vi "CreatePrivateEvents.vi"(8 "error in (no error)":errorcluster, 11 "JKI.Robot.SMO":refnum<class "JKI.Robot.SMO.lvclass">) -> (0 "error out":errorcluster, 3 "JKI.Robot.SMO out":refnum<class "JKI.Robot.SMO.lvclass">)   [LabVIEW 2014, in "JKI.Robot.SMO.lvclass"]
doc: "---------------------------------------------------------------\nJKI State Machine Objects™\nhttp://jki.net/state-machine-objects/\nCopyright (C) 2005-2015, JKI <info@jki.net>\nALL RIGHTS RESERVEDJKI State Machine Objects (SMO) 1.0.0.4\nJKI - JKI\nCopyright (c) 2015, JKI"
uses:
  JKI.Robot.SMO.lvclass
  JKI.Robot.SMO.lvclass/JKI.Robot.SMO.ctl
  Typedefs/PrivateEvents--JKI.Robot.SMO.SetGrabberPosition.ctl
  Typedefs/PrivateEvents--JKI.Robot.SMO.SetJointRotation.ctl
  Typedefs/JointType--Enum.ctl
  JKI.Robot.SMO.Base/JKI.Robot.SMO.Base.lvclass
panel:
  # "For instructions on how to use the JKI State Machine Objects, examples and video tutorials, visit:\nhttp://jki.net/state-machine-objects/\n\nJKI State Machine Objects™\nhttp://jki.net/state-machine-objects/\nCopyright (C) 2005-2015, JKI <info@jki.net>\nALL RIGHTS RESERVED"
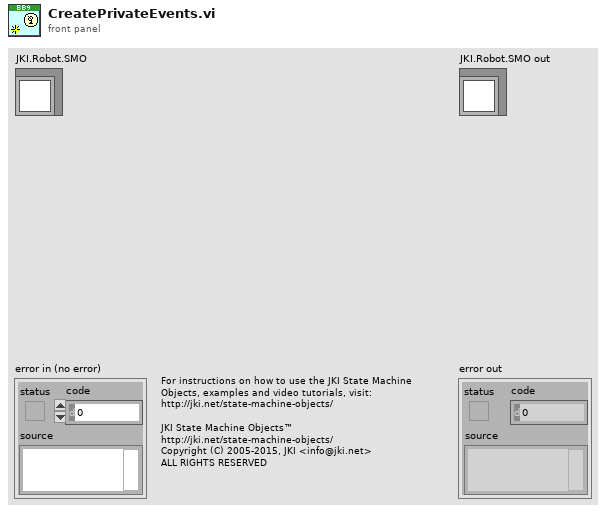
[diagram p1: front panel]
types:
  T1 = typedef "JKI.Robot.SMO.lvclass/PrivateData--Ref.ctl" = refnum<data-value>
  T2 = typedef "JKI.Robot.SMO.lvclass/PrivateEvents--JKI.Robot.SMO.SetJointRotation.ctl" = cluster{"Joint":T3, "Rotation (Deg)":dbl}
  T3 = typedef "JointType--Enum.ctl" = enum16{"A_Shoulder", "B_Elbow", "C_Wrist", "D_Base"}
  T4 = typedef "JKI.Robot.SMO.lvclass/PrivateEvents--JKI.Robot.SMO.SetGrabberPosition.ctl" = dbl
  T5 = typedef "JKI.Robot.SMO.lvclass/PrivateData--Cluster.ctl" = cluster{"Configuration":T6, "Public Events":T7, "Robot Position":T8, "Private Events":T9}
  T6 = typedef "JKI.Robot.SMO.lvclass/Configuration--Cluster.ctl" = cluster{"Suffix":string}
  T7 = typedef "JKI.Robot.SMO.lvclass/PublicEvents--Cluster.ctl" = cluster{"Data Changed":refnum<user-event>}
  T8 = typedef "RobotPosition--Cluster.ctl" = cluster{"Claw%":dbl, "JointA":dbl, "JointB":dbl, "JointC":dbl, "JointD":dbl}
  T9 = typedef "JKI.Robot.SMO.lvclass/PrivateEvents--Cluster.ctl" = cluster{"SetGrabberPosition":refnum<user-event>, "SetJointRotation":refnum<user-event>}
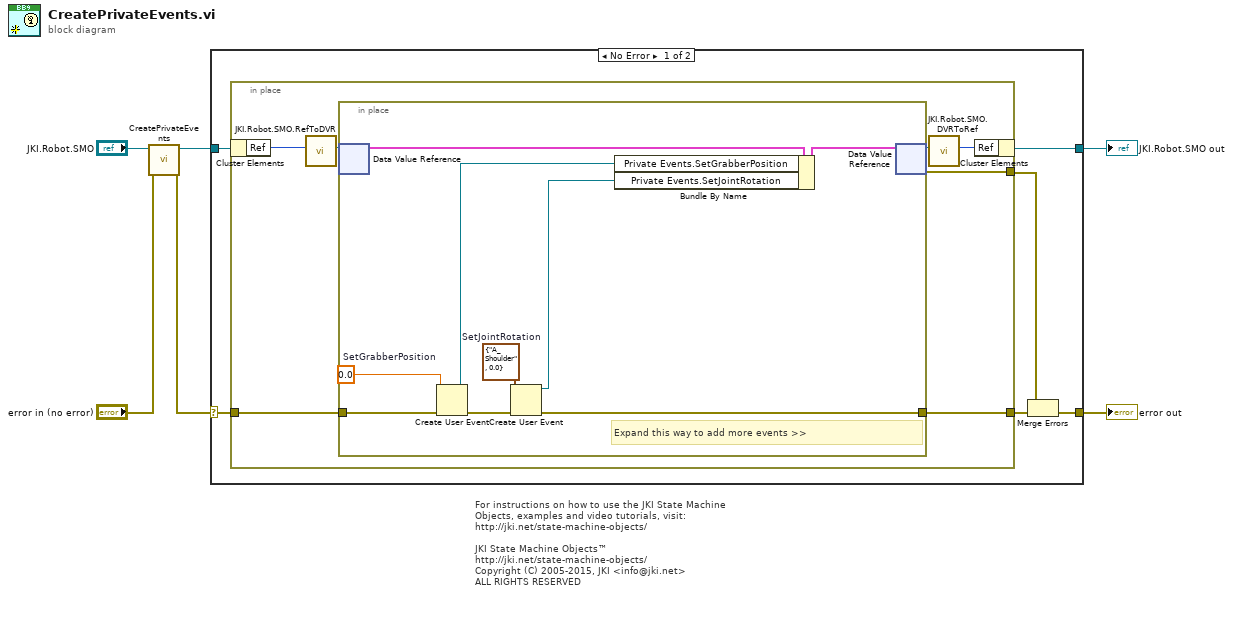
[diagram p0: block diagram]
diagram:
  # "For instructions on how to use the JKI State Machine Objects, examples and video tutorials, visit:\nhttp://jki.net/state-machine-objects/\n\nJKI State Machine Objects™\nhttp://jki.net/state-machine-objects/\nCopyright (C) 2005-2015, JKI <info@jki.net>\nALL RIGHTS RESERVED"
  n1 = call-parent "CreatePrivateEvents.vi"("error in (no error)"="error in (no error)", "SMO"="JKI.Robot.SMO") -> ("error out"=w1:errorcluster, "SMO out"=w3:refnum<class "JKI.Robot.SMO.lvclass">)  [unwired: 8 in]
  n2 = case shown="No Error" w1 {
    selector: w1 -> [w10 w30]
    tunnel: [w8 w30] -> w5
    tunnel: [w11 w29] -> w6
    tunnel: w3 -> [w12 w29]
    frame No Error {
      n3 = in-place {
        in-place-border: w10 -> [w19]
        in-place-border: [w16] -> w7
        in-place-border: [w15] -> w9
        n4 = in-place-cluster #1(w12) -> ("Ref"=w18:u32)
        n5 = call "JKI.Robot.SMO.RefToDVR.vi"("Ref"=w18) -> ("Ref"=w14:T1)  [unwired: 10 in]
        n6 = in-place {
          in-place-border: w19 -> [w28]
          in-place-border: [w22] -> w16
          w21 = T2 {"Joint"=enum."A_Shoulder", "Rotation (Deg)"=0.0}  # SetJointRotation
          w24 = T4 0.0  # SetGrabberPosition
          # "Expand this way to add more events >>"
          n7 = in-place-dvr #2(w14) -> (w27:T5)  [unwired: 1 out]
          n8 = Create User Event(user event datatype=w24, error in=w28) -> (user event=w23:refnum<user-event>, error out=w25:errorcluster)
          n9 = Create User Event(user event datatype=w21, error in=w25) -> (user event=w20:refnum<user-event>, error out=w22:errorcluster)
          n10 = Bundle By Name(cluster=w27, "Private Events.SetGrabberPosition"=w23, "Private Events.SetJointRotation"=w20) -> (w26:T5)
          n11 = in-place-dvr #2(w26) -> (w17:T1, w15:errorcluster)
        }
        n12 = call "JKI.Robot.SMO.DVRToRef.vi"("Ref"=w17) -> ("Ref"=w13:u32)  [unwired: 10 in]
        n13 = in-place-cluster #1("Ref"=w13) -> (w11:refnum<class "JKI.Robot.SMO.lvclass">)
      }
      n14 = Merge Errors(w9, w7) -> (w8:errorcluster)
    }
    frame Error {
    }
  }
  "error out" <- w5
  "JKI.Robot.SMO out" <- w6
